vi "VI Set Reentrancy.vi"(8 "error in (no error)":errorcluster, 9 "Reentrancy Type (shared clone)":T1(ring), 10 "Is Reentrant":bool, 11 "vi ref in":refnum<vi>) -> (0 "error out":errorcluster, 3 "vi ref out":refnum<vi>)   [LabVIEW 2020, in "Build Automation.lvlib"]
uses:
  Build Automation.lvlib
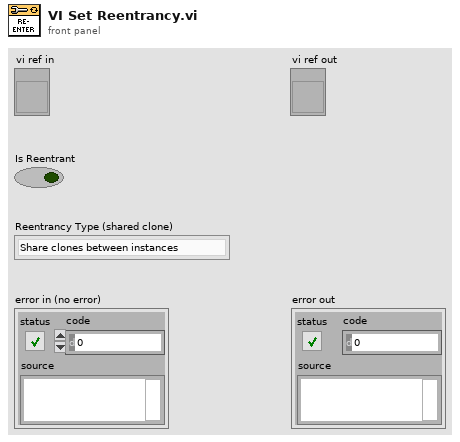
[diagram p1: front panel]
types:
  T1 = enum16{"Share clones between instances", "Preallocate clone for each instance"}
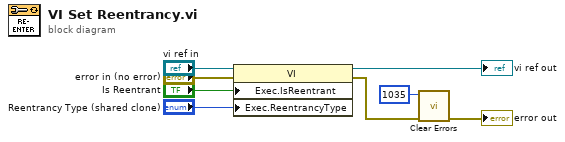
[diagram p0: block diagram]
diagram:
  n1 = property class="VI"(reference="vi ref in", error in="error in (no error)", "Exec.IsReentrant"="Is Reentrant", "Exec.ReentrancyType"="Reentrancy Type (shared clone)") -> (reference out=→"vi ref out":refnum<vi>, error out=w4:errorcluster)
  n2 = call <vilib>:"Clear Errors.vi"("error in (no error)"=w4, "specific error code to clear (0: all)"=1035) -> ("error out"=→"error out":errorcluster)  [unwired: 4 in, 1 out]
